vi "Remove NaN array1D.vi"(10 "Array in":dbl[](array[numeric])=[nan, 1.0, nan, 2.0, nan, 3.0, nan, 4.0]) -> (2 "Array out":dbl[](array[numeric]))   [LabVIEW 2016]
doc: "Removes NaN in array."
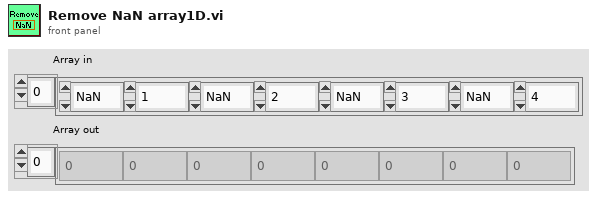
[diagram p1: front panel]
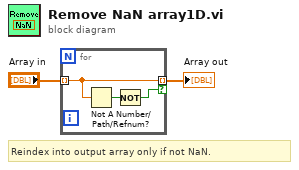
[diagram p0: block diagram]
diagram:
  # "Reindex into output array only if not NaN."
  n1 = for {
    tunnel: "Array in" -> [w5] mode=indexing
    tunnel: [w5] -> w1 mode=indexing if=w3
    n2 = Not A Number/Path/Refnum?(number/path/refnum=w5) -> (NaN/Path/Refnum?=w4:bool)
    n3 = Not(x=w4) -> (.not. x?=w3:bool)
  }
  "Array out" <- w1
